vi "to string.vi"(8 "error in":errorcluster, 11 "bin datalogger configuration in":refnum<class "Binary datalogger configuration.lvclass">) -> (0 "error out":errorcluster, 1 "data":string, 2 "version":string, 3 "bin datalogger configuration out":refnum<class "Binary datalogger configuration.lvclass">)   [LabVIEW 2013, in "Binary datalogger configuration.lvclass"]
doc: "Provides an interface for saving a module configuration to a file or other serialized data source. It is recommended that all children of this class store data in two sets--data required for its own initialization, and any data required for parent initialization--and that each implementation uses the <b>Call Parent Method</b> primitive to serialize parent information."
uses:
  Binary datalogger configuration.lvclass
  <vilib>/NI/Tag Bus Module Framework/module configuration/TBM module configuration.lvclass
  Binary datalogger configuration.lvclass/Binary datalogger configuration.ctl
  <vilib>/NI/Configuration Framework/serializable configuration/NISE_CEF_serializable configuration.lvclass
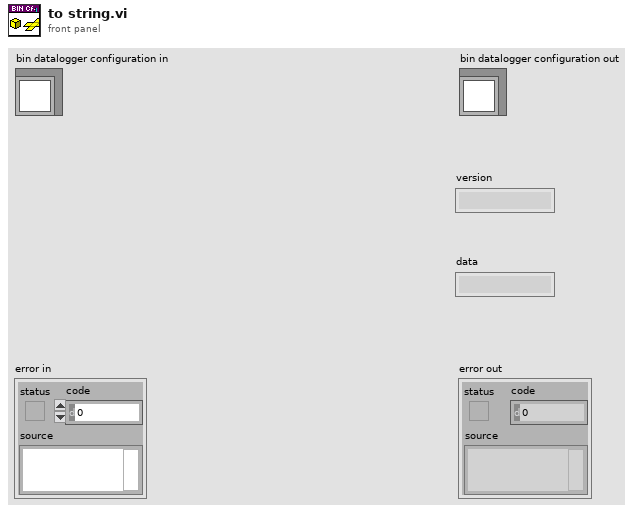
[diagram p1: front panel]
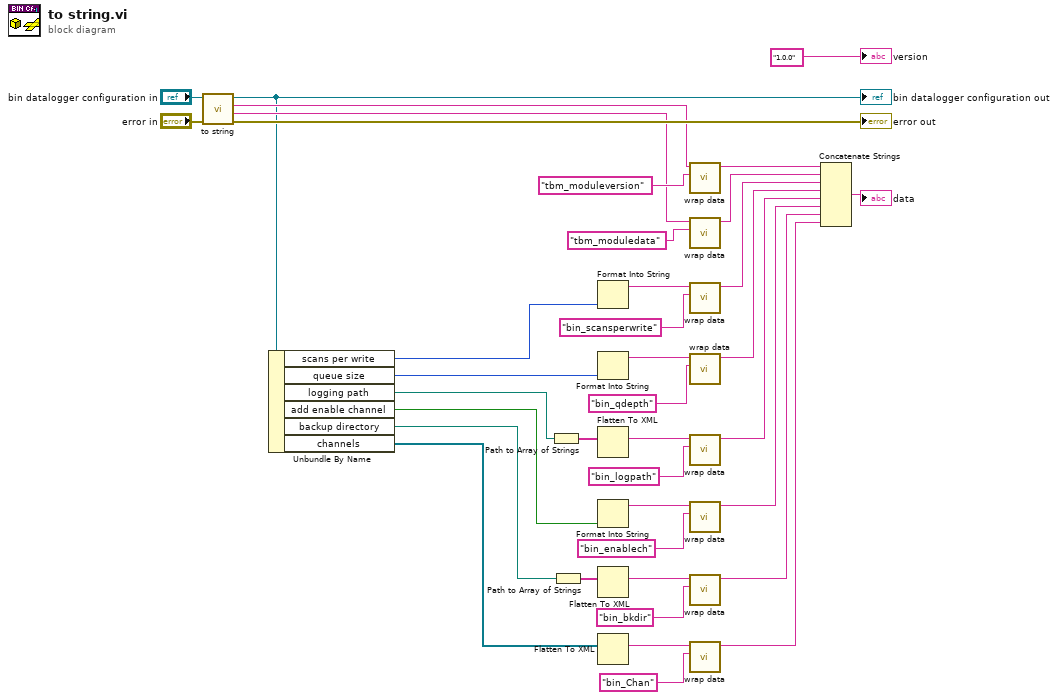
[diagram p0: block diagram]
diagram:
  n1 = call-parent "to string.vi"("error in"="error in", "module configuration in"="bin datalogger configuration in") -> ("error out"=→"error out":errorcluster, "data"=w32:string, "version"=w33:string, "module configuration out"=w28:refnum<class "Binary datalogger configuration.lvclass">)  [unwired: 6 in]
  "bin datalogger configuration out" <- w28
  n2 = Unbundle By Name(w28) -> ("scans per write"=w20:u16, "queue size"=w21:u16, "logging path"=w24:path, "add enable channel"=w22:bool, "backup directory"=w26:path, "channels"=w27:refnum<class "TBM channel.lvclass">[])
  n3 = Path to Array of Strings(0:w24) -> (2:w23:string[])  [unwired: 1 out]
  n4 = Path to Array of Strings(0:w26) -> (2:w25:string[])  [unwired: 1 out]
  n5 = Format Into String(w20) -> (resulting string=w19:string)  [unwired: 3 in, 1 out]
  n6 = Format Into String(w21) -> (resulting string=w17:string)  [unwired: 3 in, 1 out]
  n7 = Flatten To XML(anything=w23) -> (xml string=w15:string)
  n8 = Format Into String(w22) -> (resulting string=w14:string)  [unwired: 3 in, 1 out]
  n9 = Flatten To XML(anything=w25) -> (xml string=w13:string)
  n10 = Flatten To XML(anything=w27) -> (xml string=w12:string)
  n11 = call <vilib>:"wrap data.vi"("identifier"="tbm_moduleversion" ("additional identifier"), "data to wrap"=w33) -> ("wrapped data"=w31:string)  [unwired: 9 in]
  n12 = call <vilib>:"wrap data.vi"("identifier"="tbm_moduledata" ("additional identifier"), "data to wrap"=w32) -> ("wrapped data"=w29:string)  [unwired: 9 in]
  n13 = call <vilib>:"wrap data.vi"("identifier"="bin_scansperwrite" ("additional identifier"), "data to wrap"=w19) -> ("wrapped data"=w18:string)  [unwired: 9 in]
  n14 = call <vilib>:"wrap data.vi"("identifier"="bin_qdepth" ("additional identifier"), "data to wrap"=w17) -> ("wrapped data"=w16:string)  [unwired: 9 in]
  n15 = call <vilib>:"wrap data.vi"("identifier"="bin_logpath" ("additional identifier"), "data to wrap"=w15) -> ("wrapped data"=w11:string)  [unwired: 9 in]
  n16 = call <vilib>:"wrap data.vi"("identifier"="bin_enablech" ("additional identifier"), "data to wrap"=w14) -> ("wrapped data"=w10:string)  [unwired: 9 in]
  n17 = call <vilib>:"wrap data.vi"("identifier"="bin_bkdir" ("additional identifier"), "data to wrap"=w13) -> ("wrapped data"=w9:string)  [unwired: 9 in]
  n18 = call <vilib>:"wrap data.vi"("identifier"="bin_Chan" ("additional identifier"), "data to wrap"=w12) -> ("wrapped data"=w8:string)  [unwired: 9 in]
  n19 = Concatenate Strings(w31, w29, w18, w16, w11, w10, w9, w8) -> (→"data":string)
  "version" <- "1.0.0" ("current version")
